vi "RollingCurrentReadout.vi"(4 "settling\ndelay":i32, 6 "Base/High Voltage?":enum16{"Base voltage", "High voltage"}(ring), 7 "Current Threshold [nA]":dbl, 8 "disabled channels IN":i32[](array[numeric]), 9 "Flag IN":i32[](array[numeric]), 10 "Current Array IN [nA]":dbl[](array[numeric])) -> (0 "disabled channels OUT":i32[](array[numeric]), 1 "Flag OUT":i32[](array[numeric]), 3 "Current Array OUT [nA]":dbl[](array[numeric]), 5 "Compliance exceeded":bool)   [LabVIEW 2019]
doc: "Switching through channels connected to a Probe Card"
uses:
  general_VIs/globals/QC_MeasurementSetup.vi
  InstrControl/Switching/Switching.lvclass
  InstrControl/SupplyControl/SupplyControl.lvclass
panel:
  out "Display MUX":bool[][](array[boolean])
  out "Pinhole Flag":i32
  in  "last channel completed":i32
  # "Pickering Multiplexer Settings"
  # "X1"
  # "X2"
  # "X3"
  # "X4"
  # "X5"
  # "X6"
  # "X7"
  # "X8"
  # "Y1  Y2  Y3  Y4"
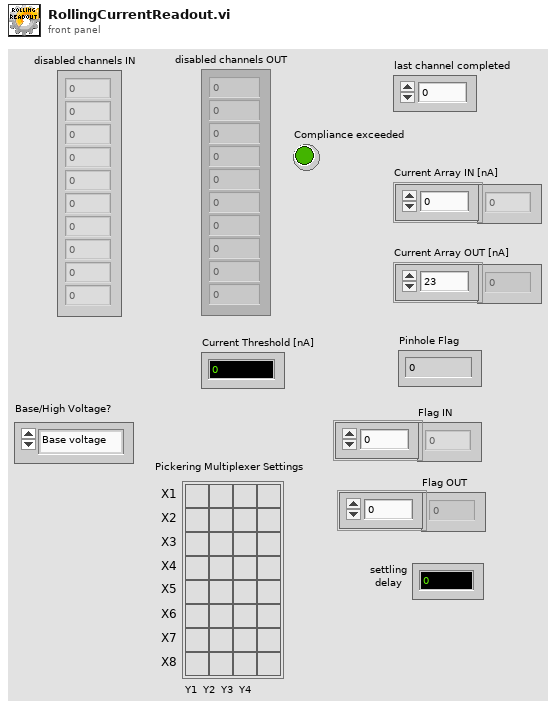
[diagram p1: front panel]
types:
  T1 = cluster{"Bias Supply":refnum<class "SupplyControl.lvclass">, "SMU":refnum<class "SupplyControl.lvclass">, "LCR":refnum<class "LCRControl.lvclass">, "Probe Card Channels":i32, "Bias Voltage [V]":dbl, "First strip":i32, "Last strip":i32, "Base Voltage [V]":dbl, "Base Ramp Step [V]":dbl, "Base Ramp Interval [ms]":u32, "High Voltage [V]":dbl, "High Ramp Step [V]":dbl, "High Ramp Interval [ms]":u32, "AC frequency [Hz]":i32, "AC amplitude [V]":dbl, "RC Configuration":u16, "Single Needle":bool, "Temperature Readout":enum16{"Read Arduino", "Enter manually"}, "Arduino":refnum<class "ArduinoControl.lvclass">, "Fraction of good strips [%]":dbl, "ProbeStation":refnum<class "ProbeStationControl.lvclass">, "Switching":refnum<class "Switching.lvclass">, "Matrix used?":bool, "Matrix X Channels":cluster{"Bias Supply / SMU LO":i32, "Bias Supply / SMU HI":i32, "CV Box LO":i32, "CV Box HI":i32, "CV Box LO IN":i32, "CV Box HI IN":i32, "Volt meter LO":i32, "Volt meter HI":i32, "Mux1 C1":i32, "Mux1 C2":i32, "Mux2 C1":i32, "Mux2 C2":i32}, "Pinholes Y/N":bool, "Capacitance Y/N":bool, "Resistance Y/N":bool, "Bias Supply Name":string, "SMU Name":string, "LCR Name":string}
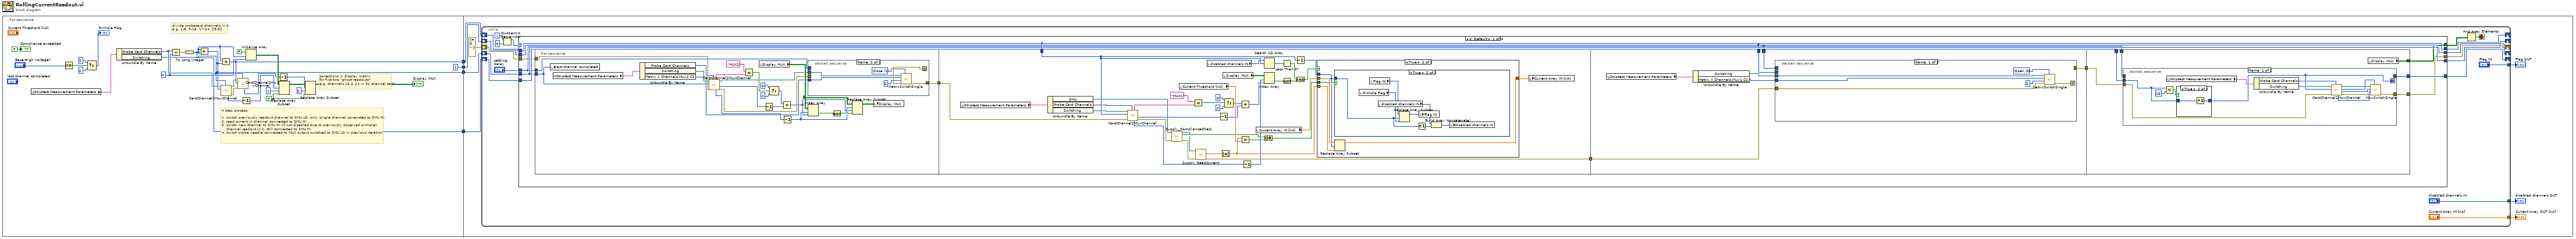
[diagram p0: block diagram]
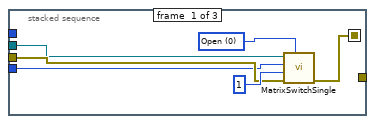
[diagram p2: hidden frame]
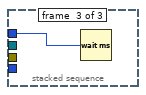
[diagram p3: hidden frame]
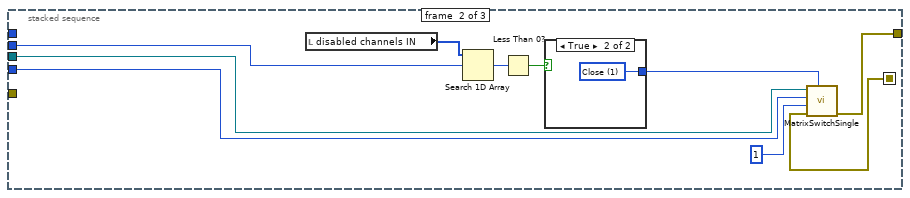
[diagram p6: hidden frame]
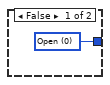
[diagram p7: hidden frame]
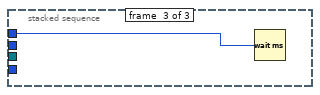
[diagram p8: hidden frame]
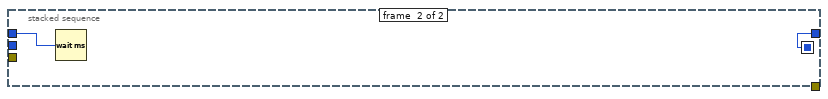
[diagram p10: hidden frame]
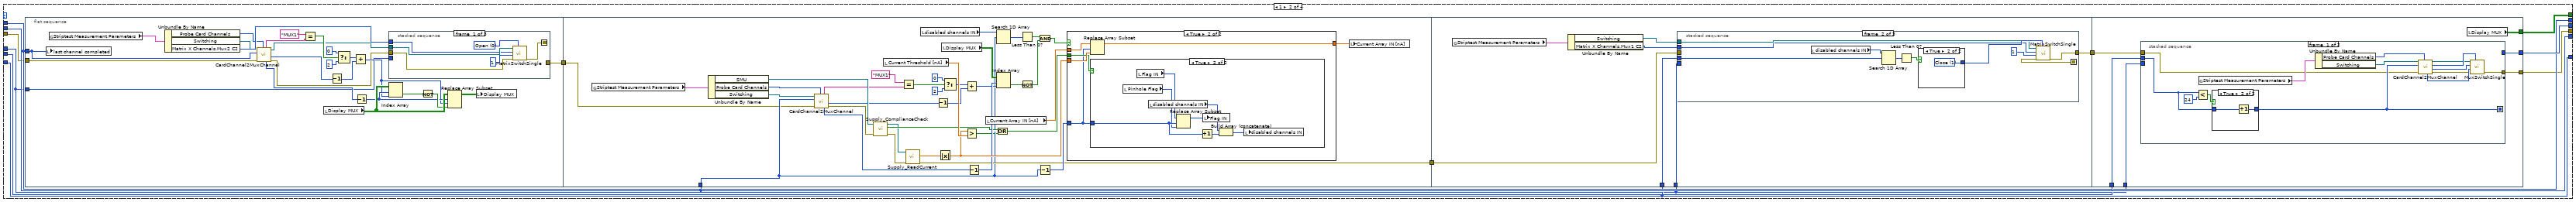
[diagram p11: hidden frame]
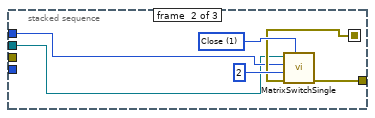
[diagram p12: hidden frame]
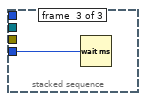
[diagram p13: hidden frame]
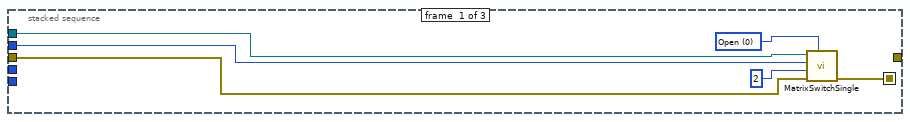
[diagram p16: hidden frame]
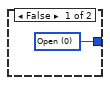
[diagram p17: hidden frame]
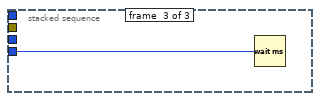
[diagram p18: hidden frame]
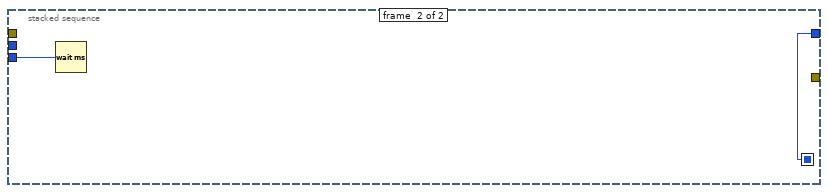
[diagram p20: hidden frame]
diagram:
  n1 = flat-sequence {
    tunnel: [1] -> w4
    tunnel: [w18] -> w3
    tunnel: [w17] -> w2
    tunnel: [w16] -> w1
    tunnel: w4 -> [w40]
    tunnel: w3 -> [w39]
    tunnel: w2 -> [w38]
    tunnel: w1 -> [w37]
    frame #0 {
      w20 = TRUE
      w30 = 4
      # "divide probecard channels in 4\ne.g. 1-8, 9-16, 17-24, 25-32"
      # "corrections in display matrix\nfor first two \"ghost readouts\"\ne.g. channels 16 & 24 in 32 channel card"
      # "4 step process:\n\n1. switch previously readout channel to SMU LO, only single channel conencted to SMU HI\n2. read current in channel connected to SMU HI\n3. switch new channel to SMU HI (if not disabled due to previously observed pinhole),\n    channel readout in 2. still connected to SMU HI\n4. switch probe needle connected to MUX output switched to SMU LO in previous iteration"
      n2 = global read "QC_MeasurementSetup.vi" "Striptest Measurement Parameters"() -> (w15:T1)
      n3 = Equal To 0?(x="Base/High Voltage?") -> (x = 0?=w11:bool)
      n4 = Select(t=1, s=w11, f=2) -> (s? t:f=→"Pinhole Flag":i32)
      n5 = Unbundle By Name(w15) -> ("Probe Card Channels"=w6:i32, "Switching"=w8:refnum<class "Switching.lvclass">)
      n6 = Divide(x=w6, y=w30) -> (x/y=w32:dbl)
      n7 = To Long Integer(number=w32) -> (32bit integer=w18:i32)
      n8 = Add(x=w18, y=w18) -> (x+y=w16:i32)
      n9 = Add(x=w18, y=w16) -> (x+y=w17:i32)
      n10 = call-dynamic "CardChannel2MuxChannel.vi"("Probe Card Channels"=w6, "Probecard Channel No."=w16, "Switching in"=w8) -> ("error out"=w5:errorcluster, "Switching out"=w7:refnum<class "Switching.lvclass">, "Channel"=w22:i32)  [unwired: 3 in, 3 out]
      n11 = call-dynamic "CardChannel2MuxChannel.vi"("Probe Card Channels"=w6, "error in (no error)"=w5, "Probecard Channel No."=w17, "Switching in"=w7) -> ("Channel"=w21:i32)  [unwired: 2 in, 5 out]
      n12 = Decrement(x=w22) -> (x-1=w28:i32)
      n13 = Initialize Array(FALSE, w18, w30) -> (w29:bool[][])
      n14 = Decrement(x=w21) -> (x-1=w25:i32)
      n15 = Replace Array Subset(array=w29, new element=w20, index (row)=w28, index (col)=1) -> (w24:bool[][])
      n16 = Replace Array Subset(array=w24, new element=w20, index (row)=w25, index (col)=2) -> (→"Display MUX":bool[][])
      "Compliance exceeded" <- FALSE
    }
    frame #1 {
      n17 = while {
        shift-right: [w52] -> _
        shift-left: w38 -> [w55]
        shift-right: [w50] -> _
        shift-left: w37 -> [w53]
        shift-right: [w51] -> _
        shift-left: w39 -> [w54]
        shift-right: [w49] -> _
        shift-left: w40 -> [w59]
        tunnel: ["disabled channels IN"] -> w34
        tunnel: ["Current Array IN [nA]"] -> w35
        tunnel: ["Flag IN"] -> w36
        shift-right: [w42] -> _
        shift-left: errorcluster {"status"=FALSE, "code"=0, "source"=""} ("error constant") -> [w41]
        i -> [w56]
        stop <- w44 stop-if-true
        n18 = Quotient & Remainder(x=w56, y=4) -> (x-y*floor(x/y)=w57:i32)  [unwired: 1 out]
        n19 = case shown="0, Default" w57 {
          tunnel: w59 -> [w67 w222 w373 w523]
          tunnel: w55 -> [w70 w219 w372 w520]
          tunnel: w54 -> [w71 w218 w370 w521]
          tunnel: w53 -> [w68 w220 w369 w522]
          tunnel: [w70 w219 w371 w520] -> w52
          tunnel: [w69 w218 w370 w521] -> w51
          tunnel: [w68 w221 w369 w522] -> w50
          tunnel: [w67 w222 w373 w524] -> w49
          tunnel: [w60 w211 w362 w513] -> w45
          tunnel: "settling\ndelay" -> [w66 w217 w368 w518]
          tunnel: [w64 w214 w365 w515] -> w42
          tunnel: w41 -> [w61 w212 w363 w514]
          frame 0, Default {
            n20 = flat-sequence {
              tunnel: w68 -> [w91]
              tunnel: w66 -> [w89]
              tunnel: [w88] -> w65
              tunnel: w61 -> [w74]
              tunnel: w70 -> [w118]
              tunnel: w65 -> [w115]
              tunnel: [w129] -> w62
              tunnel: w67 -> [w166]
              tunnel: w66 -> [w165]
              tunnel: [w164] -> w63
              tunnel: w62 -> [w163]
              tunnel: w71 -> [w191]
              tunnel: [w190] -> w69
              tunnel: w66 -> [w189]
              tunnel: [w188] -> w64
              tunnel: w63 -> [w187]
              tunnel: [w186] -> w60
              frame #0 {
                n21 = local write "last channel completed"(w91) -> ()
                n22 = global read "QC_MeasurementSetup.vi" "Striptest Measurement Parameters"() -> (w77:T1)
                n23 = Unbundle By Name(w77) -> ("Probe Card Channels"=w72:i32, "Switching"=w76:refnum<class "Switching.lvclass">, "Matrix X Channels.Mux2 C1"=w87:i32)
                n24 = call-dynamic "CardChannel2MuxChannel.vi"("Probe Card Channels"=w72, "error in (no error)"=w74, "Probecard Channel No."=w91, "Switching in"=w76) -> ("error out"=w73:errorcluster, "C1 / C2"=w80:i32, "Switching out"=w75:refnum<class "Switching.lvclass">, "Channel"=w95:i32, "Mux No. string"=w82:string)  [unwired: 2 in, 1 out]
                n25 = Equal?(x="MUX1", y=w82) -> (x = y?=w85:bool)
                n26 = local read "Display MUX"() -> (w96:bool[][])
                n27 = Decrement(x=w80) -> (x-1=w79:i32)
                n28 = Select(t=0, s=w85, f=2) -> (s? t:f=w81:i32)
                n29 = Add(x=w81, y=w79) -> (x+y=w78:i32)
                n30 = Decrement(x=w95) -> (x-1=w92:i32)
                n31 = stacked-sequence {
                  seq-local: [w100 _ _] -> [_ w106 _]
                  tunnel: [_ w105 _] -> w88
                  tunnel: w89 -> [_ _ w109]
                  tunnel: w73 -> [w99 _ _]
                  tunnel: w75 -> [w98 w104 _]
                  tunnel: w87 -> [w97 w103 _]
                  frame #0 {
                    w102 = u16 0 items=["Open", "Close"] ("Switch action")
                    n32 = call-dynamic "MatrixSwitchSingle.vi"("Switch action"=w102, "error in (no error)"=w99, "Matrix Y"=1, "Matrix X"=w97, "Switching in"=w98) -> ("error out"=w100:errorcluster)  [unwired: 4 in, 2 out]
                  }
                  frame #1 {
                    w108 = u16 1 items=["Open", "Close"] ("Switch action")
                    n33 = call-dynamic "MatrixSwitchSingle.vi"("Switch action"=w108, "error in (no error)"=w106, "Matrix Y"=2, "Matrix X"=w103, "Switching in"=w104) -> ("error out"=w105:errorcluster)  [unwired: 4 in, 2 out]
                  }
                  frame #2 {
                    n34 = Wait (ms)(milliseconds to wait=w109) -> ()  [unwired: 1 out]
                  }
                }
                n35 = Index Array(array=w96, index (row)=w92, index (col)=w78) -> (element=w94:bool)
                n36 = Not(x=w94) -> (.not. x?=w93:bool)
                n37 = Replace Array Subset(array=w96, new element=w93, index (row)=w92, index (col)=w78) -> (w90:bool[][])
                n38 = local write "Display MUX"(w90) -> ()
              }
              frame #1 {
                n39 = global read "QC_MeasurementSetup.vi" "Striptest Measurement Parameters"() -> (w116:T1)
                n40 = Unbundle By Name(w116) -> ("SMU"=w131:refnum<class "SupplyControl.lvclass">, "Probe Card Channels"=w112:i32, "Switching"=w113:refnum<class "Switching.lvclass">)
                n41 = call-dynamic "CardChannel2MuxChannel.vi"("Probe Card Channels"=w112, "error in (no error)"=w115, "Probecard Channel No."=w118, "Switching in"=w113) -> ("error out"=w114:errorcluster, "C1 / C2"=w122:i32, "Channel"=w120:i32, "Mux No. string"=w121:string)  [unwired: 2 in, 2 out]
                n42 = call-dynamic "Supply_ComplianceCheck.vi"("error in (no error)"=w114, "SupplyControl in"=w131) -> ("error out"=w146:errorcluster, "Compliance exceeded?"=w132:bool, "SupplyControl out"=w130:refnum<class "SupplyControl.lvclass">)  [unwired: 6 in, 1 out]
                n43 = local read "Current Threshold [nA]"() -> (w143:dbl)
                n44 = Equal?(x="MUX1", y=w121) -> (x = y?=w127:bool)
                n45 = call-dynamic "Supply_ReadCurrent.vi"("error in (no error)"=w146, "SupplyControl in"=w130) -> ("error out"=w129:errorcluster, "Current in nA"=w145:dbl)  [unwired: 7 in, 1 out]
                n46 = local read "disabled channels IN"() -> (w117:i32[])
                n47 = Decrement(x=w122) -> (x-1=w123:i32)
                n48 = Absolute Value(x=w145) -> (abs(x)=w144:dbl)
                n49 = local read "Display MUX"() -> (w136:bool[][])
                n50 = Select(t=0, s=w127, f=2) -> (s? t:f=w124:i32)
                n51 = Add(x=w124, y=w123) -> (x+y=w119:i32)
                n52 = Greater?(x=w144, y=w143) -> (0:w111:bool)
                n53 = Decrement(x=w120) -> (x-1=w137:i32)
                n54 = local read "Current Array IN [nA]"() -> (w142:dbl[])
                n55 = Or(x=w132, y=w111) -> (x .or. y?=w110:bool)
                n56 = Search 1D Array(1D array=w117, element=w118) -> (index of element=w140:i32)  [unwired: 1 in]
                n57 = Index Array(array=w136, index (row)=w137, index (col)=w119) -> (element=w138:bool)
                n58 = Less Than 0?(x=w140) -> (x < 0?=w135:bool)
                n59 = Not(x=w138) -> (.not. x?=w134:bool)
                n60 = Decrement(x=w118) -> (x-1=w139:i32)
                n61 = And(x=w135, y=w134) -> (x .and. y?=w133:bool)
                n62 = case shown="True" w133 {
                  tunnel: w144 -> [_ w152]
                  tunnel: w142 -> [w147 w151]
                  tunnel: [w147 w150] -> w141
                  tunnel: w139 -> [_ w148]
                  tunnel: w110 -> [_ w149]
                  frame False {
                  }
                  frame True {
                    n63 = case shown="True" w149 {
                      tunnel: w148 -> [_ w156]
                      frame False {
                      }
                      frame True {
                        n64 = local read "Pinhole Flag"() -> (w153:i32)
                        n65 = local read "Flag IN"() -> (w159:i32[])
                        n66 = local read "disabled channels IN"() -> (w157:i32[])
                        n67 = Replace Array Subset(array=w159, new element=w153, index=w156) -> (w158:i32[])
                        n68 = Increment(x=w156) -> (x+1=w155:i32)
                        n69 = local write "Flag IN"(w158) -> ()
                        n70 = Build Array (concatenate)(w157, w155) -> (w154:i32[])
                        n71 = local write "disabled channels IN"(w154) -> ()
                      }
                    }
                    n72 = Replace Array Subset(array=w151, new element=w152, index=w148) -> (w150:dbl[])
                  }
                }
                n73 = local write "Current Array IN [nA]"(w141) -> ()
              }
              frame #2 {
                n74 = global read "QC_MeasurementSetup.vi" "Striptest Measurement Parameters"() -> (w160:T1)
                n75 = Unbundle By Name(w160) -> ("Switching"=w162:refnum<class "Switching.lvclass">, "Matrix X Channels.Mux1 C1"=w161:i32)
                n76 = stacked-sequence {
                  seq-local: [w170 _ _] -> [_ w176 _]
                  tunnel: w166 -> [_ w178 _]
                  tunnel: [_ w177 _] -> w164
                  tunnel: w165 -> [_ _ w185]
                  tunnel: w163 -> [w169 _ _]
                  tunnel: w162 -> [w168 w175 _]
                  tunnel: w161 -> [w167 w174 _]
                  frame #0 {
                    w171 = u16 0 items=["Open", "Close"] ("Switch action")
                    n77 = call-dynamic "MatrixSwitchSingle.vi"("Switch action"=w171, "error in (no error)"=w169, "Matrix Y"=2, "Matrix X"=w167, "Switching in"=w168) -> ("error out"=w170:errorcluster)  [unwired: 4 in, 2 out]
                  }
                  frame #1 {
                    n78 = local read "disabled channels IN"() -> (w173:i32[])
                    n79 = Search 1D Array(1D array=w173, element=w178) -> (index of element=w180:i32)  [unwired: 1 in]
                    n80 = Less Than 0?(x=w180) -> (x < 0?=w181:bool)
                    n81 = case shown="True" w181 {
                      tunnel: [w183 w184] -> w179
                      frame False {
                        w183 = u16 0 items=["Open", "Close"] ("Switch action")
                      }
                      frame True {
                        w184 = u16 1 items=["Open", "Close"] ("Switch action")
                      }
                    }
                    n82 = call-dynamic "MatrixSwitchSingle.vi"("Switch action"=w179, "error in (no error)"=w176, "Matrix Y"=1, "Matrix X"=w174, "Switching in"=w175) -> ("error out"=w177:errorcluster)  [unwired: 4 in, 2 out]
                  }
                  frame #2 {
                    n83 = Wait (ms)(milliseconds to wait=w185) -> ()  [unwired: 1 out]
                  }
                }
              }
              frame #3 {
                n84 = stacked-sequence {
                  seq-local: [w199 _] -> [_ w210]
                  tunnel: w191 -> [w201 _]
                  tunnel: [w198 _] -> w188
                  tunnel: w187 -> [w194 _]
                  tunnel: [_ w210] -> w190
                  tunnel: w189 -> [_ w209]
                  frame #0 {
                    n85 = Less?(x=w201, y=16) -> (x < y?=w202:bool)
                    n86 = global read "QC_MeasurementSetup.vi" "Striptest Measurement Parameters"() -> (w197:T1)
                    n87 = case shown="True" w202 {
                      tunnel: w201 -> [w206 w208]
                      tunnel: [w206 w207] -> w199
                      frame False {
                      }
                      frame True {
                        n88 = Increment(x=w208) -> (x+1=w207:i32)
                      }
                    }
                    n89 = Unbundle By Name(w197) -> ("Probe Card Channels"=w192:i32, "Switching"=w196:refnum<class "Switching.lvclass">)
                    n90 = call-dynamic "CardChannel2MuxChannel.vi"("Probe Card Channels"=w192, "error in (no error)"=w194, "Probecard Channel No."=w199, "Switching in"=w196) -> ("error out"=w193:errorcluster, "C1 / C2"=w204:i32, "Mux No.:"=w203:u32, "Switching out"=w195:refnum<class "Switching.lvclass">, "Channel"=w205:i32)  [unwired: 2 in, 1 out]
                    n91 = call-dynamic "MuxSwitchSingle.vi"("MUX address"=w203, "error in (no error)"=w193, "Channel"=w205, "C1 / C2"=w204, "Switching in"=w195) -> ("error out"=w198:errorcluster)  [unwired: 4 in, 2 out]
                  }
                  frame #1 {
                    n92 = Wait (ms)(milliseconds to wait=w209) -> ()  [unwired: 1 out]
                  }
                }
                n93 = local read "Display MUX"() -> (w186:bool[][])
              }
            }
          }
          frame 1 {
            n94 = flat-sequence {
              tunnel: w219 -> [w242]
              tunnel: w217 -> [w240]
              tunnel: [w239] -> w216
              tunnel: w212 -> [w226]
              tunnel: w222 -> [w269]
              tunnel: w216 -> [w265]
              tunnel: [w280] -> w213
              tunnel: w218 -> [w317]
              tunnel: w217 -> [w316]
              tunnel: [w315] -> w215
              tunnel: w213 -> [w314]
              tunnel: w220 -> [w342]
              tunnel: [w341] -> w221
              tunnel: w217 -> [w340]
              tunnel: w215 -> [w339]
              tunnel: [w338] -> w214
              tunnel: [w337] -> w211
              frame #0 {
                n95 = local write "last channel completed"(w242) -> ()
                n96 = global read "QC_MeasurementSetup.vi" "Striptest Measurement Parameters"() -> (w228:T1)
                n97 = Unbundle By Name(w228) -> ("Probe Card Channels"=w224:i32, "Switching"=w227:refnum<class "Switching.lvclass">, "Matrix X Channels.Mux2 C2"=w238:i32)
                n98 = call-dynamic "CardChannel2MuxChannel.vi"("Probe Card Channels"=w224, "error in (no error)"=w226, "Probecard Channel No."=w242, "Switching in"=w227) -> ("error out"=w225:errorcluster, "C1 / C2"=w229:i32, "Switching out"=w223:refnum<class "Switching.lvclass">, "Channel"=w246:i32, "Mux No. string"=w231:string)  [unwired: 2 in, 1 out]
                n99 = Equal?(x="MUX1", y=w231) -> (x = y?=w236:bool)
                n100 = local read "Display MUX"() -> (w247:bool[][])
                n101 = Decrement(x=w229) -> (x-1=w232:i32)
                n102 = Select(t=0, s=w236, f=2) -> (s? t:f=w233:i32)
                n103 = Add(x=w233, y=w232) -> (x+y=w230:i32)
                n104 = Decrement(x=w246) -> (x-1=w243:i32)
                n105 = stacked-sequence {
                  seq-local: [w251 _ _] -> [_ w257 _]
                  tunnel: [_ w256 _] -> w239
                  tunnel: w240 -> [_ _ w260]
                  tunnel: w225 -> [w250 _ _]
                  tunnel: w223 -> [w249 w254 _]
                  tunnel: w238 -> [w248 w255 _]
                  frame #0 {
                    w253 = u16 0 items=["Open", "Close"] ("Switch action")
                    n106 = call-dynamic "MatrixSwitchSingle.vi"("Switch action"=w253, "error in (no error)"=w250, "Matrix Y"=1, "Matrix X"=w248, "Switching in"=w249) -> ("error out"=w251:errorcluster)  [unwired: 4 in, 2 out]
                  }
                  frame #1 {
                    w259 = u16 1 items=["Open", "Close"] ("Switch action")
                    n107 = call-dynamic "MatrixSwitchSingle.vi"("Switch action"=w259, "error in (no error)"=w257, "Matrix Y"=2, "Matrix X"=w255, "Switching in"=w254) -> ("error out"=w256:errorcluster)  [unwired: 4 in, 2 out]
                  }
                  frame #2 {
                    n108 = Wait (ms)(milliseconds to wait=w260) -> ()  [unwired: 1 out]
                  }
                }
                n109 = Index Array(array=w247, index (row)=w243, index (col)=w230) -> (element=w245:bool)
                n110 = Not(x=w245) -> (.not. x?=w244:bool)
                n111 = Replace Array Subset(array=w247, new element=w244, index (row)=w243, index (col)=w230) -> (w241:bool[][])
                n112 = local write "Display MUX"(w241) -> ()
              }
              frame #1 {
                n113 = global read "QC_MeasurementSetup.vi" "Striptest Measurement Parameters"() -> (w267:T1)
                n114 = Unbundle By Name(w267) -> ("SMU"=w282:refnum<class "SupplyControl.lvclass">, "Probe Card Channels"=w263:i32, "Switching"=w266:refnum<class "Switching.lvclass">)
                n115 = call-dynamic "CardChannel2MuxChannel.vi"("Probe Card Channels"=w263, "error in (no error)"=w265, "Probecard Channel No."=w269, "Switching in"=w266) -> ("error out"=w264:errorcluster, "C1 / C2"=w273:i32, "Channel"=w271:i32, "Mux No. string"=w272:string)  [unwired: 2 in, 2 out]
                n116 = call-dynamic "Supply_ComplianceCheck.vi"("error in (no error)"=w264, "SupplyControl in"=w282) -> ("error out"=w297:errorcluster, "Compliance exceeded?"=w283:bool, "SupplyControl out"=w281:refnum<class "SupplyControl.lvclass">)  [unwired: 6 in, 1 out]
                n117 = local read "Current Threshold [nA]"() -> (w295:dbl)
                n118 = Equal?(x="MUX1", y=w272) -> (x = y?=w278:bool)
                n119 = call-dynamic "Supply_ReadCurrent.vi"("error in (no error)"=w297, "SupplyControl in"=w281) -> ("error out"=w280:errorcluster, "Current in nA"=w296:dbl)  [unwired: 7 in, 1 out]
                n120 = local read "disabled channels IN"() -> (w268:i32[])
                n121 = Decrement(x=w273) -> (x-1=w274:i32)
                n122 = Absolute Value(x=w296) -> (abs(x)=w292:dbl)
                n123 = local read "Display MUX"() -> (w287:bool[][])
                n124 = Select(t=0, s=w278, f=2) -> (s? t:f=w275:i32)
                n125 = Add(x=w275, y=w274) -> (x+y=w270:i32)
                n126 = Greater?(x=w292, y=w295) -> (0:w262:bool)
                n127 = Decrement(x=w271) -> (x-1=w288:i32)
                n128 = local read "Current Array IN [nA]"() -> (w294:dbl[])
                n129 = Or(x=w283, y=w262) -> (x .or. y?=w261:bool)
                n130 = Search 1D Array(1D array=w268, element=w269) -> (index of element=w291:i32)  [unwired: 1 in]
                n131 = Index Array(array=w287, index (row)=w288, index (col)=w270) -> (element=w289:bool)
                n132 = Less Than 0?(x=w291) -> (x < 0?=w286:bool)
                n133 = Not(x=w289) -> (.not. x?=w285:bool)
                n134 = And(x=w286, y=w285) -> (x .and. y?=w284:bool)
                n135 = Decrement(x=w269) -> (x-1=w290:i32)
                n136 = case shown="True" w284 {
                  tunnel: w294 -> [w298 w303]
                  tunnel: [w298 w302] -> w293
                  tunnel: w290 -> [_ w299]
                  tunnel: w292 -> [_ w301]
                  tunnel: w261 -> [_ w300]
                  frame False {
                  }
                  frame True {
                    n137 = Replace Array Subset(array=w303, new element=w301, index=w299) -> (w302:dbl[])
                    n138 = case shown="True" w300 {
                      tunnel: w299 -> [_ w307]
                      frame False {
                      }
                      frame True {
                        n139 = local read "Pinhole Flag"() -> (w304:i32)
                        n140 = local read "Flag IN"() -> (w310:i32[])
                        n141 = local read "disabled channels IN"() -> (w308:i32[])
                        n142 = Replace Array Subset(array=w310, new element=w304, index=w307) -> (w309:i32[])
                        n143 = Increment(x=w307) -> (x+1=w306:i32)
                        n144 = local write "Flag IN"(w309) -> ()
                        n145 = Build Array (concatenate)(w308, w306) -> (w305:i32[])
                        n146 = local write "disabled channels IN"(w305) -> ()
                      }
                    }
                  }
                }
                n147 = local write "Current Array IN [nA]"(w293) -> ()
              }
              frame #2 {
                n148 = global read "QC_MeasurementSetup.vi" "Striptest Measurement Parameters"() -> (w311:T1)
                n149 = Unbundle By Name(w311) -> ("Switching"=w313:refnum<class "Switching.lvclass">, "Matrix X Channels.Mux1 C2"=w312:i32)
                n150 = stacked-sequence {
                  seq-local: [w321 _ _] -> [_ w328 _]
                  tunnel: w317 -> [_ w329 _]
                  tunnel: [_ w327 _] -> w315
                  tunnel: w316 -> [_ _ w336]
                  tunnel: w314 -> [w320 _ _]
                  tunnel: w313 -> [w319 w326 _]
                  tunnel: w312 -> [w318 w325 _]
                  frame #0 {
                    w322 = u16 0 items=["Open", "Close"] ("Switch action")
                    n151 = call-dynamic "MatrixSwitchSingle.vi"("Switch action"=w322, "error in (no error)"=w320, "Matrix Y"=2, "Matrix X"=w318, "Switching in"=w319) -> ("error out"=w321:errorcluster)  [unwired: 4 in, 2 out]
                  }
                  frame #1 {
                    n152 = local read "disabled channels IN"() -> (w324:i32[])
                    n153 = Search 1D Array(1D array=w324, element=w329) -> (index of element=w330:i32)  [unwired: 1 in]
                    n154 = Less Than 0?(x=w330) -> (x < 0?=w331:bool)
                    n155 = case shown="True" w331 {
                      tunnel: [w334 w335] -> w332
                      frame False {
                        w334 = u16 0 items=["Open", "Close"] ("Switch action")
                      }
                      frame True {
                        w335 = u16 1 items=["Open", "Close"] ("Switch action")
                      }
                    }
                    n156 = call-dynamic "MatrixSwitchSingle.vi"("Switch action"=w332, "error in (no error)"=w328, "Matrix Y"=1, "Matrix X"=w325, "Switching in"=w326) -> ("error out"=w327:errorcluster)  [unwired: 4 in, 2 out]
                  }
                  frame #2 {
                    n157 = Wait (ms)(milliseconds to wait=w336) -> ()  [unwired: 1 out]
                  }
                }
              }
              frame #3 {
                n158 = stacked-sequence {
                  seq-local: [w350 _] -> [_ w361]
                  tunnel: w342 -> [w351 _]
                  tunnel: w339 -> [w345 _]
                  tunnel: [_ w361] -> w341
                  tunnel: w340 -> [_ w360]
                  tunnel: [w349 _] -> w338
                  frame #0 {
                    n159 = Less?(x=w351, y=24) -> (x < y?=w353:bool)
                    n160 = global read "QC_MeasurementSetup.vi" "Striptest Measurement Parameters"() -> (w348:T1)
                    n161 = case shown="True" w353 {
                      tunnel: w351 -> [w357 w359]
                      tunnel: [w357 w358] -> w350
                      frame False {
                      }
                      frame True {
                        n162 = Increment(x=w359) -> (x+1=w358:i32)
                      }
                    }
                    n163 = Unbundle By Name(w348) -> ("Probe Card Channels"=w343:i32, "Switching"=w347:refnum<class "Switching.lvclass">)
                    n164 = call-dynamic "CardChannel2MuxChannel.vi"("Probe Card Channels"=w343, "error in (no error)"=w345, "Probecard Channel No."=w350, "Switching in"=w347) -> ("error out"=w344:errorcluster, "C1 / C2"=w355:i32, "Mux No.:"=w354:u32, "Switching out"=w346:refnum<class "Switching.lvclass">, "Channel"=w356:i32)  [unwired: 2 in, 1 out]
                    n165 = call-dynamic "MuxSwitchSingle.vi"("MUX address"=w354, "error in (no error)"=w344, "Channel"=w356, "C1 / C2"=w355, "Switching in"=w346) -> ("error out"=w349:errorcluster)  [unwired: 4 in, 2 out]
                  }
                  frame #1 {
                    n166 = Wait (ms)(milliseconds to wait=w360) -> ()  [unwired: 1 out]
                  }
                }
                n167 = local read "Display MUX"() -> (w337:bool[][])
              }
            }
          }
          frame 2 {
            n168 = flat-sequence {
              tunnel: w373 -> [w398]
              tunnel: w368 -> [w391]
              tunnel: [w390] -> w367
              tunnel: w363 -> [w375]
              tunnel: w370 -> [w419]
              tunnel: w367 -> [w414]
              tunnel: [w430] -> w364
              tunnel: w369 -> [w468]
              tunnel: w368 -> [w467]
              tunnel: [w466] -> w366
              tunnel: w364 -> [w465]
              tunnel: w372 -> [w493]
              tunnel: [w492] -> w371
              tunnel: w368 -> [w491]
              tunnel: w366 -> [w490]
              tunnel: [w489] -> w365
              tunnel: [w488] -> w362
              frame #0 {
                n169 = local write "last channel completed"(w398) -> ()
                n170 = global read "QC_MeasurementSetup.vi" "Striptest Measurement Parameters"() -> (w379:T1)
                n171 = Unbundle By Name(w379) -> ("Probe Card Channels"=w378:i32, "Switching"=w377:refnum<class "Switching.lvclass">, "Matrix X Channels.Mux1 C1"=w389:i32)
                n172 = call-dynamic "CardChannel2MuxChannel.vi"("Probe Card Channels"=w378, "error in (no error)"=w375, "Probecard Channel No."=w398, "Switching in"=w377) -> ("error out"=w374:errorcluster, "C1 / C2"=w382:i32, "Switching out"=w376:refnum<class "Switching.lvclass">, "Channel"=w397:i32, "Mux No. string"=w381:string)  [unwired: 2 in, 1 out]
                n173 = Equal?(x="MUX1", y=w381) -> (x = y?=w387:bool)
                n174 = local read "Display MUX"() -> (w394:bool[][])
                n175 = Decrement(x=w382) -> (x-1=w383:i32)
                n176 = Select(t=0, s=w387, f=2) -> (s? t:f=w384:i32)
                n177 = Add(x=w384, y=w383) -> (x+y=w380:i32)
                n178 = Decrement(x=w397) -> (x-1=w393:i32)
                n179 = Index Array(array=w394, index (row)=w393, index (col)=w380) -> (element=w396:bool)
                n180 = stacked-sequence {
                  seq-local: [w402 _ _] -> [_ w408 _]
                  tunnel: w374 -> [w401 _ _]
                  tunnel: [_ w407 _] -> w390
                  tunnel: w391 -> [_ _ w411]
                  tunnel: w376 -> [w400 w406 _]
                  tunnel: w389 -> [w399 w405 _]
                  frame #0 {
                    w404 = u16 0 items=["Open", "Close"] ("Switch action")
                    n181 = call-dynamic "MatrixSwitchSingle.vi"("Switch action"=w404, "error in (no error)"=w401, "Matrix Y"=1, "Matrix X"=w399, "Switching in"=w400) -> ("error out"=w402:errorcluster)  [unwired: 4 in, 2 out]
                  }
                  frame #1 {
                    w410 = u16 1 items=["Open", "Close"] ("Switch action")
                    n182 = call-dynamic "MatrixSwitchSingle.vi"("Switch action"=w410, "error in (no error)"=w408, "Matrix Y"=2, "Matrix X"=w405, "Switching in"=w406) -> ("error out"=w407:errorcluster)  [unwired: 4 in, 2 out]
                  }
                  frame #2 {
                    n183 = Wait (ms)(milliseconds to wait=w411) -> ()  [unwired: 1 out]
                  }
                }
                n184 = Not(x=w396) -> (.not. x?=w395:bool)
                n185 = Replace Array Subset(array=w394, new element=w395, index (row)=w393, index (col)=w380) -> (w392:bool[][])
                n186 = local write "Display MUX"(w392) -> ()
              }
              frame #1 {
                n187 = global read "QC_MeasurementSetup.vi" "Striptest Measurement Parameters"() -> (w433:T1)
                n188 = Unbundle By Name(w433) -> ("SMU"=w432:refnum<class "SupplyControl.lvclass">, "Probe Card Channels"=w416:i32, "Switching"=w417:refnum<class "Switching.lvclass">)
                n189 = call-dynamic "CardChannel2MuxChannel.vi"("Probe Card Channels"=w416, "error in (no error)"=w414, "Probecard Channel No."=w419, "Switching in"=w417) -> ("error out"=w415:errorcluster, "C1 / C2"=w423:i32, "Channel"=w420:i32, "Mux No. string"=w422:string)  [unwired: 2 in, 2 out]
                n190 = call-dynamic "Supply_ComplianceCheck.vi"("error in (no error)"=w415, "SupplyControl in"=w432) -> ("error out"=w448:errorcluster, "Compliance exceeded?"=w434:bool, "SupplyControl out"=w431:refnum<class "SupplyControl.lvclass">)  [unwired: 6 in, 1 out]
                n191 = local read "Current Threshold [nA]"() -> (w446:dbl)
                n192 = Equal?(x="MUX1", y=w422) -> (x = y?=w428:bool)
                n193 = call-dynamic "Supply_ReadCurrent.vi"("error in (no error)"=w448, "SupplyControl in"=w431) -> ("error out"=w430:errorcluster, "Current in nA"=w447:dbl)  [unwired: 7 in, 1 out]
                n194 = local read "disabled channels IN"() -> (w418:i32[])
                n195 = Decrement(x=w423) -> (x-1=w424:i32)
                n196 = Absolute Value(x=w447) -> (abs(x)=w443:dbl)
                n197 = local read "Display MUX"() -> (w439:bool[][])
                n198 = Select(t=0, s=w428, f=2) -> (s? t:f=w425:i32)
                n199 = Add(x=w425, y=w424) -> (x+y=w421:i32)
                n200 = Greater?(x=w443, y=w446) -> (0:w413:bool)
                n201 = Decrement(x=w420) -> (x-1=w440:i32)
                n202 = local read "Current Array IN [nA]"() -> (w445:dbl[])
                n203 = Or(x=w434, y=w413) -> (x .or. y?=w412:bool)
                n204 = Index Array(array=w439, index (row)=w440, index (col)=w421) -> (element=w436:bool)
                n205 = Search 1D Array(1D array=w418, element=w419) -> (index of element=w442:i32)  [unwired: 1 in]
                n206 = Not(x=w436) -> (.not. x?=w435:bool)
                n207 = Less Than 0?(x=w442) -> (x < 0?=w438:bool)
                n208 = And(x=w438, y=w435) -> (x .and. y?=w437:bool)
                n209 = Decrement(x=w419) -> (x-1=w441:i32)
                n210 = case shown="True" w437 {
                  tunnel: w443 -> [_ w454]
                  tunnel: w445 -> [w449 w453]
                  tunnel: [w449 w452] -> w444
                  tunnel: w441 -> [_ w451]
                  tunnel: w412 -> [_ w450]
                  frame False {
                  }
                  frame True {
                    n211 = Replace Array Subset(array=w453, new element=w454, index=w451) -> (w452:dbl[])
                    n212 = case shown="True" w450 {
                      tunnel: w451 -> [_ w458]
                      frame False {
                      }
                      frame True {
                        n213 = local read "Pinhole Flag"() -> (w455:i32)
                        n214 = local read "Flag IN"() -> (w461:i32[])
                        n215 = local read "disabled channels IN"() -> (w459:i32[])
                        n216 = Replace Array Subset(array=w461, new element=w455, index=w458) -> (w460:i32[])
                        n217 = Increment(x=w458) -> (x+1=w457:i32)
                        n218 = local write "Flag IN"(w460) -> ()
                        n219 = Build Array (concatenate)(w459, w457) -> (w456:i32[])
                        n220 = local write "disabled channels IN"(w456) -> ()
                      }
                    }
                  }
                }
                n221 = local write "Current Array IN [nA]"(w444) -> ()
              }
              frame #2 {
                n222 = global read "QC_MeasurementSetup.vi" "Striptest Measurement Parameters"() -> (w462:T1)
                n223 = Unbundle By Name(w462) -> ("Switching"=w464:refnum<class "Switching.lvclass">, "Matrix X Channels.Mux2 C1"=w463:i32)
                n224 = stacked-sequence {
                  seq-local: [w472 _ _] -> [_ w478 _]
                  tunnel: w465 -> [w471 _ _]
                  tunnel: w468 -> [_ w480 _]
                  tunnel: [_ w479 _] -> w466
                  tunnel: w467 -> [_ _ w487]
                  tunnel: w464 -> [w470 w477 _]
                  tunnel: w463 -> [w469 w476 _]
                  frame #0 {
                    w473 = u16 0 items=["Open", "Close"] ("Switch action")
                    n225 = call-dynamic "MatrixSwitchSingle.vi"("Switch action"=w473, "error in (no error)"=w471, "Matrix Y"=2, "Matrix X"=w469, "Switching in"=w470) -> ("error out"=w472:errorcluster)  [unwired: 4 in, 2 out]
                  }
                  frame #1 {
                    n226 = local read "disabled channels IN"() -> (w475:i32[])
                    n227 = Search 1D Array(1D array=w475, element=w480) -> (index of element=w482:i32)  [unwired: 1 in]
                    n228 = Less Than 0?(x=w482) -> (x < 0?=w483:bool)
                    n229 = case shown="True" w483 {
                      tunnel: [w485 w486] -> w481
                      frame False {
                        w485 = u16 0 items=["Open", "Close"] ("Switch action")
                      }
                      frame True {
                        w486 = u16 1 items=["Open", "Close"] ("Switch action")
                      }
                    }
                    n230 = call-dynamic "MatrixSwitchSingle.vi"("Switch action"=w481, "error in (no error)"=w478, "Matrix Y"=1, "Matrix X"=w476, "Switching in"=w477) -> ("error out"=w479:errorcluster)  [unwired: 4 in, 2 out]
                  }
                  frame #2 {
                    n231 = Wait (ms)(milliseconds to wait=w487) -> ()  [unwired: 1 out]
                  }
                }
              }
              frame #3 {
                n232 = stacked-sequence {
                  seq-local: [w501 _] -> [_ w512]
                  tunnel: w493 -> [w502 _]
                  tunnel: w490 -> [w494 _]
                  tunnel: [w500 _] -> w489
                  tunnel: [_ w512] -> w492
                  tunnel: w491 -> [_ w511]
                  frame #0 {
                    n233 = Less?(x=w502, y=32) -> (x < y?=w504:bool)
                    n234 = global read "QC_MeasurementSetup.vi" "Striptest Measurement Parameters"() -> (w499:T1)
                    n235 = case shown="True" w504 {
                      tunnel: w502 -> [w508 w510]
                      tunnel: [w508 w509] -> w501
                      frame False {
                      }
                      frame True {
                        n236 = Increment(x=w510) -> (x+1=w509:i32)
                      }
                    }
                    n237 = Unbundle By Name(w499) -> ("Probe Card Channels"=w498:i32, "Switching"=w497:refnum<class "Switching.lvclass">)
                    n238 = call-dynamic "CardChannel2MuxChannel.vi"("Probe Card Channels"=w498, "error in (no error)"=w494, "Probecard Channel No."=w501, "Switching in"=w497) -> ("error out"=w496:errorcluster, "C1 / C2"=w506:i32, "Mux No.:"=w505:u32, "Switching out"=w495:refnum<class "Switching.lvclass">, "Channel"=w507:i32)  [unwired: 2 in, 1 out]
                    n239 = call-dynamic "MuxSwitchSingle.vi"("MUX address"=w505, "error in (no error)"=w496, "Channel"=w507, "C1 / C2"=w506, "Switching in"=w495) -> ("error out"=w500:errorcluster)  [unwired: 4 in, 2 out]
                  }
                  frame #1 {
                    n240 = Wait (ms)(milliseconds to wait=w511) -> ()  [unwired: 1 out]
                  }
                }
                n241 = local read "Display MUX"() -> (w488:bool[][])
              }
            }
          }
          frame 3 {
            n242 = flat-sequence {
              tunnel: w521 -> [w545]
              tunnel: w518 -> [w542]
              tunnel: [w541] -> w519
              tunnel: w514 -> [w528]
              tunnel: w522 -> [w573]
              tunnel: w519 -> [w567]
              tunnel: [w582] -> w517
              tunnel: w520 -> [w620]
              tunnel: w518 -> [w619]
              tunnel: w517 -> [w618]
              tunnel: [w617] -> w516
              tunnel: w523 -> [w645]
              tunnel: [w644] -> w524
              tunnel: w518 -> [w643]
              tunnel: w516 -> [w642]
              tunnel: [w641] -> w515
              tunnel: [w640] -> w513
              frame #0 {
                n243 = local write "last channel completed"(w545) -> ()
                n244 = global read "QC_MeasurementSetup.vi" "Striptest Measurement Parameters"() -> (w530:T1)
                n245 = Unbundle By Name(w530) -> ("Probe Card Channels"=w529:i32, "Switching"=w526:refnum<class "Switching.lvclass">, "Matrix X Channels.Mux1 C2"=w540:i32)
                n246 = call-dynamic "CardChannel2MuxChannel.vi"("Probe Card Channels"=w529, "error in (no error)"=w528, "Probecard Channel No."=w545, "Switching in"=w526) -> ("error out"=w527:errorcluster, "C1 / C2"=w533:i32, "Switching out"=w525:refnum<class "Switching.lvclass">, "Channel"=w550:i32, "Mux No. string"=w531:string)  [unwired: 2 in, 1 out]
                n247 = Equal?(x="MUX1", y=w531) -> (x = y?=w538:bool)
                n248 = Decrement(x=w533) -> (x-1=w534:i32)
                n249 = Select(t=0, s=w538, f=2) -> (s? t:f=w535:i32)
                n250 = Add(x=w535, y=w534) -> (x+y=w532:i32)
                n251 = local read "Display MUX"() -> (w544:bool[][])
                n252 = Decrement(x=w532) -> (x-1=w547:i32)
                n253 = Decrement(x=w550) -> (x-1=w546:i32)
                n254 = stacked-sequence {
                  seq-local: [w554 _ _] -> [_ w560 _]
                  tunnel: [_ w559 _] -> w541
                  tunnel: w542 -> [_ _ w563]
                  tunnel: w527 -> [w553 _ _]
                  tunnel: w525 -> [w552 w557 _]
                  tunnel: w540 -> [w551 w558 _]
                  frame #0 {
                    w556 = u16 0 items=["Open", "Close"] ("Switch action")
                    n255 = call-dynamic "MatrixSwitchSingle.vi"("Switch action"=w556, "error in (no error)"=w553, "Matrix Y"=1, "Matrix X"=w551, "Switching in"=w552) -> ("error out"=w554:errorcluster)  [unwired: 4 in, 2 out]
                  }
                  frame #1 {
                    w562 = u16 1 items=["Open", "Close"] ("Switch action")
                    n256 = call-dynamic "MatrixSwitchSingle.vi"("Switch action"=w562, "error in (no error)"=w560, "Matrix Y"=2, "Matrix X"=w558, "Switching in"=w557) -> ("error out"=w559:errorcluster)  [unwired: 4 in, 2 out]
                  }
                  frame #2 {
                    n257 = Wait (ms)(milliseconds to wait=w563) -> ()  [unwired: 1 out]
                  }
                }
                n258 = Index Array(array=w544, index (row)=w546, index (col)=w547) -> (element=w549:bool)
                n259 = Not(x=w549) -> (.not. x?=w548:bool)
                n260 = Replace Array Subset(array=w544, new element=w548, index (row)=w546, index (col)=w547) -> (w543:bool[][])
                n261 = local write "Display MUX"(w543) -> ()
              }
              frame #1 {
                n262 = global read "QC_MeasurementSetup.vi" "Striptest Measurement Parameters"() -> (w584:T1)
                n263 = Unbundle By Name(w584) -> ("SMU"=w583:refnum<class "SupplyControl.lvclass">, "Probe Card Channels"=w568:i32, "Switching"=w569:refnum<class "Switching.lvclass">)
                n264 = call-dynamic "CardChannel2MuxChannel.vi"("Probe Card Channels"=w568, "error in (no error)"=w567, "Probecard Channel No."=w573, "Switching in"=w569) -> ("error out"=w566:errorcluster, "C1 / C2"=w575:i32, "Channel"=w572:i32, "Mux No. string"=w574:string)  [unwired: 2 in, 2 out]
                n265 = call-dynamic "Supply_ComplianceCheck.vi"("error in (no error)"=w566, "SupplyControl in"=w583) -> ("error out"=w600:errorcluster, "Compliance exceeded?"=w586:bool, "SupplyControl out"=w585:refnum<class "SupplyControl.lvclass">)  [unwired: 6 in, 1 out]
                n266 = local read "Current Threshold [nA]"() -> (w598:dbl)
                n267 = Equal?(x="MUX1", y=w574) -> (x = y?=w580:bool)
                n268 = call-dynamic "Supply_ReadCurrent.vi"("error in (no error)"=w600, "SupplyControl in"=w585) -> ("error out"=w582:errorcluster, "Current in nA"=w599:dbl)  [unwired: 7 in, 1 out]
                n269 = local read "disabled channels IN"() -> (w570:i32[])
                n270 = local read "Display MUX"() -> (w590:bool[][])
                n271 = Decrement(x=w575) -> (x-1=w576:i32)
                n272 = Absolute Value(x=w599) -> (abs(x)=w595:dbl)
                n273 = Select(t=0, s=w580, f=2) -> (s? t:f=w577:i32)
                n274 = Add(x=w577, y=w576) -> (x+y=w571:i32)
                n275 = Greater?(x=w595, y=w598) -> (0:w565:bool)
                n276 = Decrement(x=w572) -> (x-1=w591:i32)
                n277 = local read "Current Array IN [nA]"() -> (w596:dbl[])
                n278 = Or(x=w586, y=w565) -> (x .or. y?=w564:bool)
                n279 = Search 1D Array(1D array=w570, element=w573) -> (index of element=w597:i32)  [unwired: 1 in]
                n280 = Index Array(array=w590, index (row)=w591, index (col)=w571) -> (element=w592:bool)
                n281 = Less Than 0?(x=w597) -> (x < 0?=w589:bool)
                n282 = Not(x=w592) -> (.not. x?=w588:bool)
                n283 = Decrement(x=w573) -> (x-1=w593:i32)
                n284 = And(x=w589, y=w588) -> (x .and. y?=w587:bool)
                n285 = case shown="True" w587 {
                  tunnel: w595 -> [_ w606]
                  tunnel: w596 -> [w601 w605]
                  tunnel: [w601 w604] -> w594
                  tunnel: w593 -> [_ w602]
                  tunnel: w564 -> [_ w603]
                  frame False {
                  }
                  frame True {
                    n286 = Replace Array Subset(array=w605, new element=w606, index=w602) -> (w604:dbl[])
                    n287 = case shown="True" w603 {
                      tunnel: w602 -> [_ w610]
                      frame False {
                      }
                      frame True {
                        n288 = local read "Pinhole Flag"() -> (w607:i32)
                        n289 = local read "Flag IN"() -> (w613:i32[])
                        n290 = local read "disabled channels IN"() -> (w611:i32[])
                        n291 = Replace Array Subset(array=w613, new element=w607, index=w610) -> (w612:i32[])
                        n292 = Increment(x=w610) -> (x+1=w609:i32)
                        n293 = local write "Flag IN"(w612) -> ()
                        n294 = Build Array (concatenate)(w611, w609) -> (w608:i32[])
                        n295 = local write "disabled channels IN"(w608) -> ()
                      }
                    }
                  }
                }
                n296 = local write "Current Array IN [nA]"(w594) -> ()
              }
              frame #2 {
                n297 = global read "QC_MeasurementSetup.vi" "Striptest Measurement Parameters"() -> (w614:T1)
                n298 = Unbundle By Name(w614) -> ("Switching"=w616:refnum<class "Switching.lvclass">, "Matrix X Channels.Mux2 C2"=w615:i32)
                n299 = stacked-sequence {
                  seq-local: [w624 _ _] -> [_ w631 _]
                  tunnel: w618 -> [w623 _ _]
                  tunnel: w620 -> [_ w632 _]
                  tunnel: [_ w630 _] -> w617
                  tunnel: w619 -> [_ _ w639]
                  tunnel: w616 -> [w621 w629 _]
                  tunnel: w615 -> [w622 w628 _]
                  frame #0 {
                    w625 = u16 0 items=["Open", "Close"] ("Switch action")
                    n300 = call-dynamic "MatrixSwitchSingle.vi"("Switch action"=w625, "error in (no error)"=w623, "Matrix Y"=2, "Matrix X"=w622, "Switching in"=w621) -> ("error out"=w624:errorcluster)  [unwired: 4 in, 2 out]
                  }
                  frame #1 {
                    n301 = local read "disabled channels IN"() -> (w627:i32[])
                    n302 = Search 1D Array(1D array=w627, element=w632) -> (index of element=w634:i32)  [unwired: 1 in]
                    n303 = Less Than 0?(x=w634) -> (x < 0?=w635:bool)
                    n304 = case shown="True" w635 {
                      tunnel: [w637 w638] -> w633
                      frame False {
                        w637 = u16 0 items=["Open", "Close"] ("Switch action")
                      }
                      frame True {
                        w638 = u16 1 items=["Open", "Close"] ("Switch action")
                      }
                    }
                    n305 = call-dynamic "MatrixSwitchSingle.vi"("Switch action"=w633, "error in (no error)"=w631, "Matrix Y"=1, "Matrix X"=w628, "Switching in"=w629) -> ("error out"=w630:errorcluster)  [unwired: 4 in, 2 out]
                  }
                  frame #2 {
                    n306 = Wait (ms)(milliseconds to wait=w639) -> ()  [unwired: 1 out]
                  }
                }
              }
              frame #3 {
                n307 = stacked-sequence {
                  seq-local: [w653 _] -> [_ w664]
                  tunnel: w645 -> [w654 _]
                  tunnel: w642 -> [w647 _]
                  tunnel: [w652 _] -> w641
                  tunnel: [_ w664] -> w644
                  tunnel: w643 -> [_ w663]
                  frame #0 {
                    n308 = Less?(x=w654, y=8) -> (x < y?=w656:bool)
                    n309 = case shown="True" w656 {
                      tunnel: w654 -> [w660 w662]
                      tunnel: [w660 w661] -> w653
                      frame False {
                      }
                      frame True {
                        n310 = Increment(x=w662) -> (x+1=w661:i32)
                      }
                    }
                    n311 = global read "QC_MeasurementSetup.vi" "Striptest Measurement Parameters"() -> (w651:T1)
                    n312 = Unbundle By Name(w651) -> ("Probe Card Channels"=w650:i32, "Switching"=w648:refnum<class "Switching.lvclass">)
                    n313 = call-dynamic "CardChannel2MuxChannel.vi"("Probe Card Channels"=w650, "error in (no error)"=w647, "Probecard Channel No."=w653, "Switching in"=w648) -> ("error out"=w646:errorcluster, "C1 / C2"=w658:i32, "Mux No.:"=w657:u32, "Switching out"=w649:refnum<class "Switching.lvclass">, "Channel"=w659:i32)  [unwired: 2 in, 1 out]
                    n314 = call-dynamic "MuxSwitchSingle.vi"("MUX address"=w657, "error in (no error)"=w646, "Channel"=w659, "C1 / C2"=w658, "Switching in"=w649) -> ("error out"=w652:errorcluster)  [unwired: 4 in, 2 out]
                  }
                  frame #1 {
                    n315 = Wait (ms)(milliseconds to wait=w663) -> ()  [unwired: 1 out]
                  }
                }
                n316 = local read "Display MUX"() -> (w640:bool[][])
              }
            }
          }
        }
        n317 = And Array Elements(Boolean array=w45) -> (logical AND=w44:bool)
      }
      "Flag OUT" <- w36
      "Current Array OUT [nA]" <- w35
      "disabled channels OUT" <- w34
    }
  }
